vi "getArrayNotZeroIdx.vi"(8 "error in (no error)":errorcluster, 10 "Array":dbl[](array[numeric]), 11 "MatOper in":refnum<class "MatOper.lvclass">) -> (0 "error out":errorcluster, 2 "Index Array":i32[](array[numeric]), 3 "MatOper out":refnum<class "MatOper.lvclass">)   [LabVIEW 2016, in "MatOper.lvclass"]
doc: "Get the non-zero index array."
uses:
  MatOper.lvclass
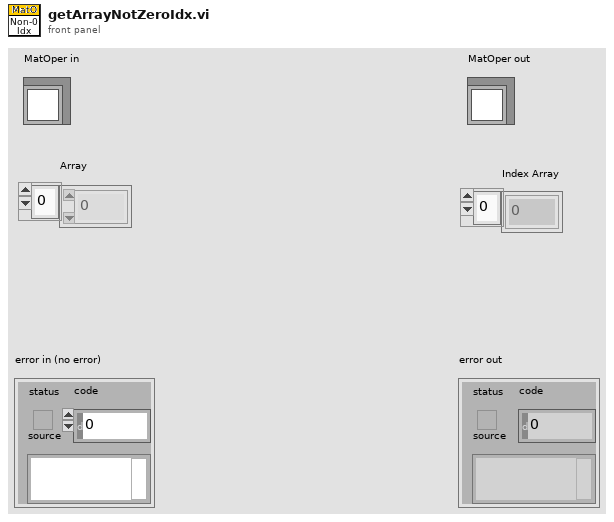
[diagram p1: front panel]
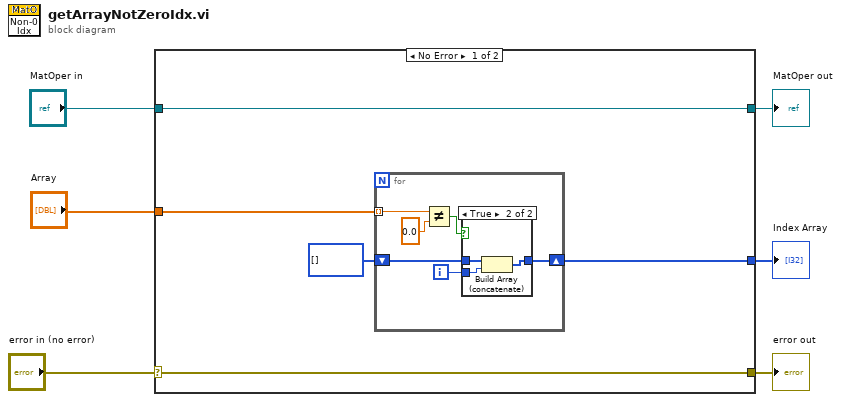
[diagram p0: block diagram]
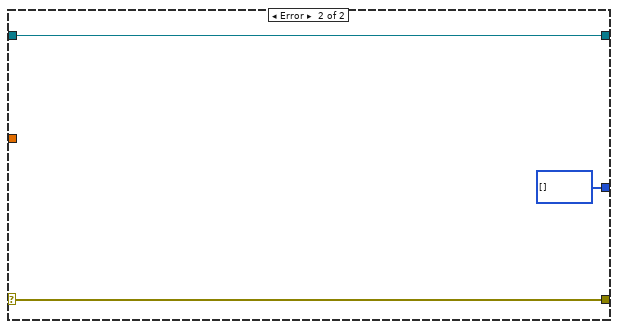
[diagram p3: hidden frame]
diagram:
  n1 = case shown="No Error" "error in (no error)" {
    selector: "error in (no error)" -> [w10 w24]
    tunnel: [w10 w24] -> w5
    tunnel: [w11 w23] -> w3
    tunnel: "MatOper in" -> [w11 w23]
    tunnel: "Array" -> [w8 _]
    tunnel: [w7 i32[] []] -> w1
    frame No Error {
      n2 = for {
        tunnel: w8 -> [w16] mode=indexing
        shift-right: [w12] -> w7
        shift-left: i32[] [] -> [w13]
        i -> [w14]
        n3 = Not Equal?(x=w16, y=0.0) -> (x != y?=w17:bool)
        n4 = case shown="True" w17 {
          tunnel: w14 -> [_ w21]
          tunnel: w13 -> [w18 w20]
          tunnel: [w18 w19] -> w12
          frame False {
          }
          frame True {
            n5 = Build Array (concatenate)(w20, w21) -> (w19:i32[])
          }
        }
      }
    }
    frame Error {
    }
  }
  "error out" <- w5
  "MatOper out" <- w3
  "Index Array" <- w1
